vi "Configure SMU Negative Voltage Limit.vi"(8 "error in (no error)":errorcluster {"code" format="%.0x"}, 9 "Negative Voltage Limit (0.0 volts)":dbl format="%^.3e", 10 "Channel Name (1)":string="1", 11 "VISA resource name":refnum<visa-resource-name>) -> (0 "error out":errorcluster {"code" format="%.0x"}, 3 "VISA resource name out":refnum<visa-resource-name>)   [LabVIEW 2016, in "Agilent N6700 Series.lvlib"]
doc: "Sets the negative voltage limit of the specified output channel.\n\n<b>Notes:</b>\n(1) This VI only applies to model N6784A.\n(2) The output protection priority must be set to current in <b>Configure Output Regulation.vi</b>."
uses:
  <instrlib>/Agilent N6700 Series/Agilent N6700 Series.lvlib
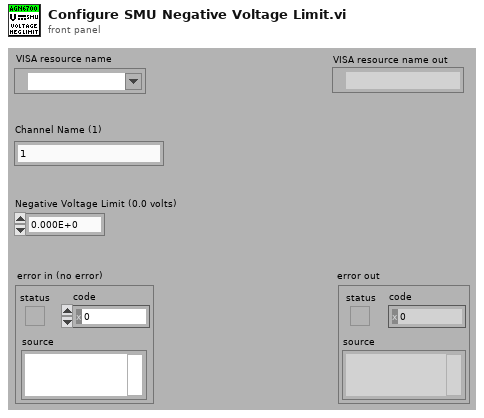
[diagram p1: front panel]
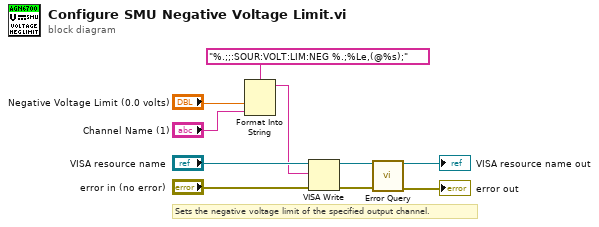
[diagram p0: block diagram]
diagram:
  # "Sets the negative voltage limit of the specified output channel."
  n1 = Format Into String(format string="%.;;:SOUR:VOLT:LIM:NEG %.;%Le,(@%s);", "Negative Voltage Limit (0.0 volts)", "Channel Name (1)") -> (resulting string=w4:string)  [unwired: 2 in, 1 out]
  n2 = VISA Write(VISA resource name="VISA resource name", write buffer=w4, error in (no error)="error in (no error)") -> (VISA resource name out=w6:refnum<visa-resource-name>, error out=w5:errorcluster)  [unwired: 1 out]
  n3 = call <instrlib>:"Error Query.vi"("VISA resource name"=w6, "error in (no error)"=w5) -> ("VISA resource name out"=→"VISA resource name out":refnum<visa-resource-name>, "error out"=→"error out":errorcluster)  [unwired: 10 in, 2 out]
